vi "Periodic Tasks.vi"(8 "error in":errorcluster) -> ()   [LabVIEW 2020]
doc: "This VI runs in parallel to other tasks. It can contain as many user-defined periodic loops as you need. These can carry out PID or other sorts of timed response."
uses:
  <vilib>/Rock Robotics/WPI/ThirdParty/Sensors/navX/_TypeDefs/FRIC_navX_DeviceNumbersTypeDef.ctl
  <vilib>/Rock Robotics/WPI/ThirdParty/JAS_Junk/TrajLib/Rotation2d_CreateAngle.vi
  Robot Global Data.vi
  <vilib>/Rock Robotics/WPI/ThirdParty/Phoenix-LabVIEW/CANCoder/Get/CTRE_Phoenix_CANcoder_GetSensorData.vi
  <vilib>/Rock Robotics/WPI/ThirdParty/JAS_Junk/TrajLib/Trajectory_Library.lvlib
  <vilib>/Rock Robotics/Network Tables/NT Write Number.vi
  <vilib>/Rock Robotics/Network Tables/NT Write Boolean.vi
panel:
  out "POSE.TRANSLATION.Y":dbl
  out "POSE.TRANSLATION.X":dbl
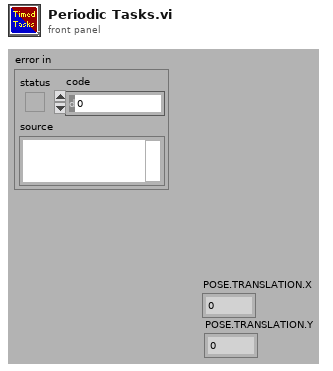
[diagram p1: front panel]
types:
  T1 = typedef "Trajectory_Library.lvlib/ROTATION2D.ctl" = cluster{"VALUE":dbl, "COS":dbl, "SIN":dbl}
  T2 = typedef "Trajectory_Library.lvlib/TRANSLATION2D.ctl" = cluster{"X":dbl, "Y":dbl}
  T3 = typedef "Trajectory_Library.lvlib/SWERVE_DRIVE_MODULE_POSITION.ctl" = cluster{"Distance":dbl, "Angle":T1, "P":bool}
  T4 = typedef "Trajectory_Library.lvlib/POSE2D.ctl" = cluster{"TRANSLATION":T2, "ROTATION":T1}
  T5 = typedef "Trajectory_Library.lvlib/SWERVE_DRIVE_KINEMATICS.ctl" = cluster{"NumModules":i32, "InverseKinematics":T6, "ForwardKinematics":T6, "Modules":T2[], "PrevCoR":T2, "SavedModuleStates":T7[]}
  T6 = typedef "NI_Matrix.lvlib/RealMatrix.ctl" = dbl[][]
  T7 = typedef "Trajectory_Library.lvlib/SWERVE_DRIVE_MODULE_STATE.ctl" = cluster{"Speed":dbl, "Angle":T1}
  T8 = typedef "Trajectory_Library.lvlib/SWERVE_DRIVE_ODOMETRY.ctl" = cluster{"POSE":T4, "GyroOffset":T1, "PreviousAngle":T1, "PrevModulePositions":T3[], "NumModules":i32}
  T9 = typedef "FRIC_navX_DeviceNumbersTypeDef.ctl" = enum16{"Dev0", "Dev1", "Dev2", "Dev3"}
  T10 = typedef "CTRE_Phoenix_CANcoder_DeviceRef.ctl" = cluster{"DeviceStatus":errorcluster, "Device Number":u8, "Handle":u64, "UsageFrame":u32, "Library Path":path}
  T11 = typedef "WPI_MotorControlDeviceRef.ctl" = cluster{"DeviceStatus":errorcluster, "Type":T12, "PWM":cluster{"PWM Channel":T13, "DeadBand":T14}, "CAN":cluster{"Device Number":u8, "SetOutput VI Ref":variant, "GetOutput VI Ref":variant, "Enable VI Ref":variant, "Disable VI Ref":variant, "Data":variant}, "Invert":bool, "DIO PWM":cluster{"PWM \"Enable\" Channel":T13, "DIOChannel":T15, "PWM Rate":dbl}}
  T12 = typedef "WPI_MotorControlType.ctl" = enum16{"PWM", "CAN", "DIO PWM"}
  T13 = typedef "FPGA_DIOPWMChannel.ctl" = enum8{"PWM 0", "PWM 1", "PWM 2", "PWM 3", "PWM 4", "PWM 5", "PWM 6", "PWM 7", "PWM 8", "PWM 9", "PWM MXP 0", "PWM MXP 1", "PWM MXP 2", "PWM MXP 3", "PWM MXP 4", "PWM MXP 5", "PWM MXP 6", "PWM MXP 7", "PWM MXP 8", "PWM MXP 9", "Invalid"}
  T14 = typedef "WPI_PWMDeadband.ctl" = cluster{"Name":string, "maxPositivePwm":i32, "minPositivePwm":i32, "centerPwm":i32, "maxNegativePwm":i32, "minNegativePwm":i32, "angularRange":u16}
  T15 = typedef "FPGA_DIOChannel.ctl" = enum8{"DIO 0", "DIO 1", "DIO 2", "DIO 3", "DIO 4", "DIO 5", "DIO 6", "DIO 7", "DIO 8", "DIO 9", "DIO MXP 0", "DIO MXP 1", "DIO MXP 2", "DIO MXP 3", "DIO MXP 4", "DIO MXP 5", "DIO MXP 6", "DIO MXP 7", "DIO MXP 8", "DIO MXP 9", "DIO MXP 10", "DIO MXP 11", "DIO MXP 12", "DIO MXP 13", "DIO MXP 14", "DIO MXP 15", "SPI Port CS1", "SPI Port CS2", "SPI Port CS3", "SPI Port MISO", "SPI Port MOSI", "Invalid"}
  T16 = cluster{"Yaw":dbl, "Roll":dbl, "Pitch":dbl, "Heading":dbl, "Fused Heading":dbl}
  T17 = cluster{"POSE.TRANSLATION.X":dbl, "POSE.TRANSLATION.Y":dbl}
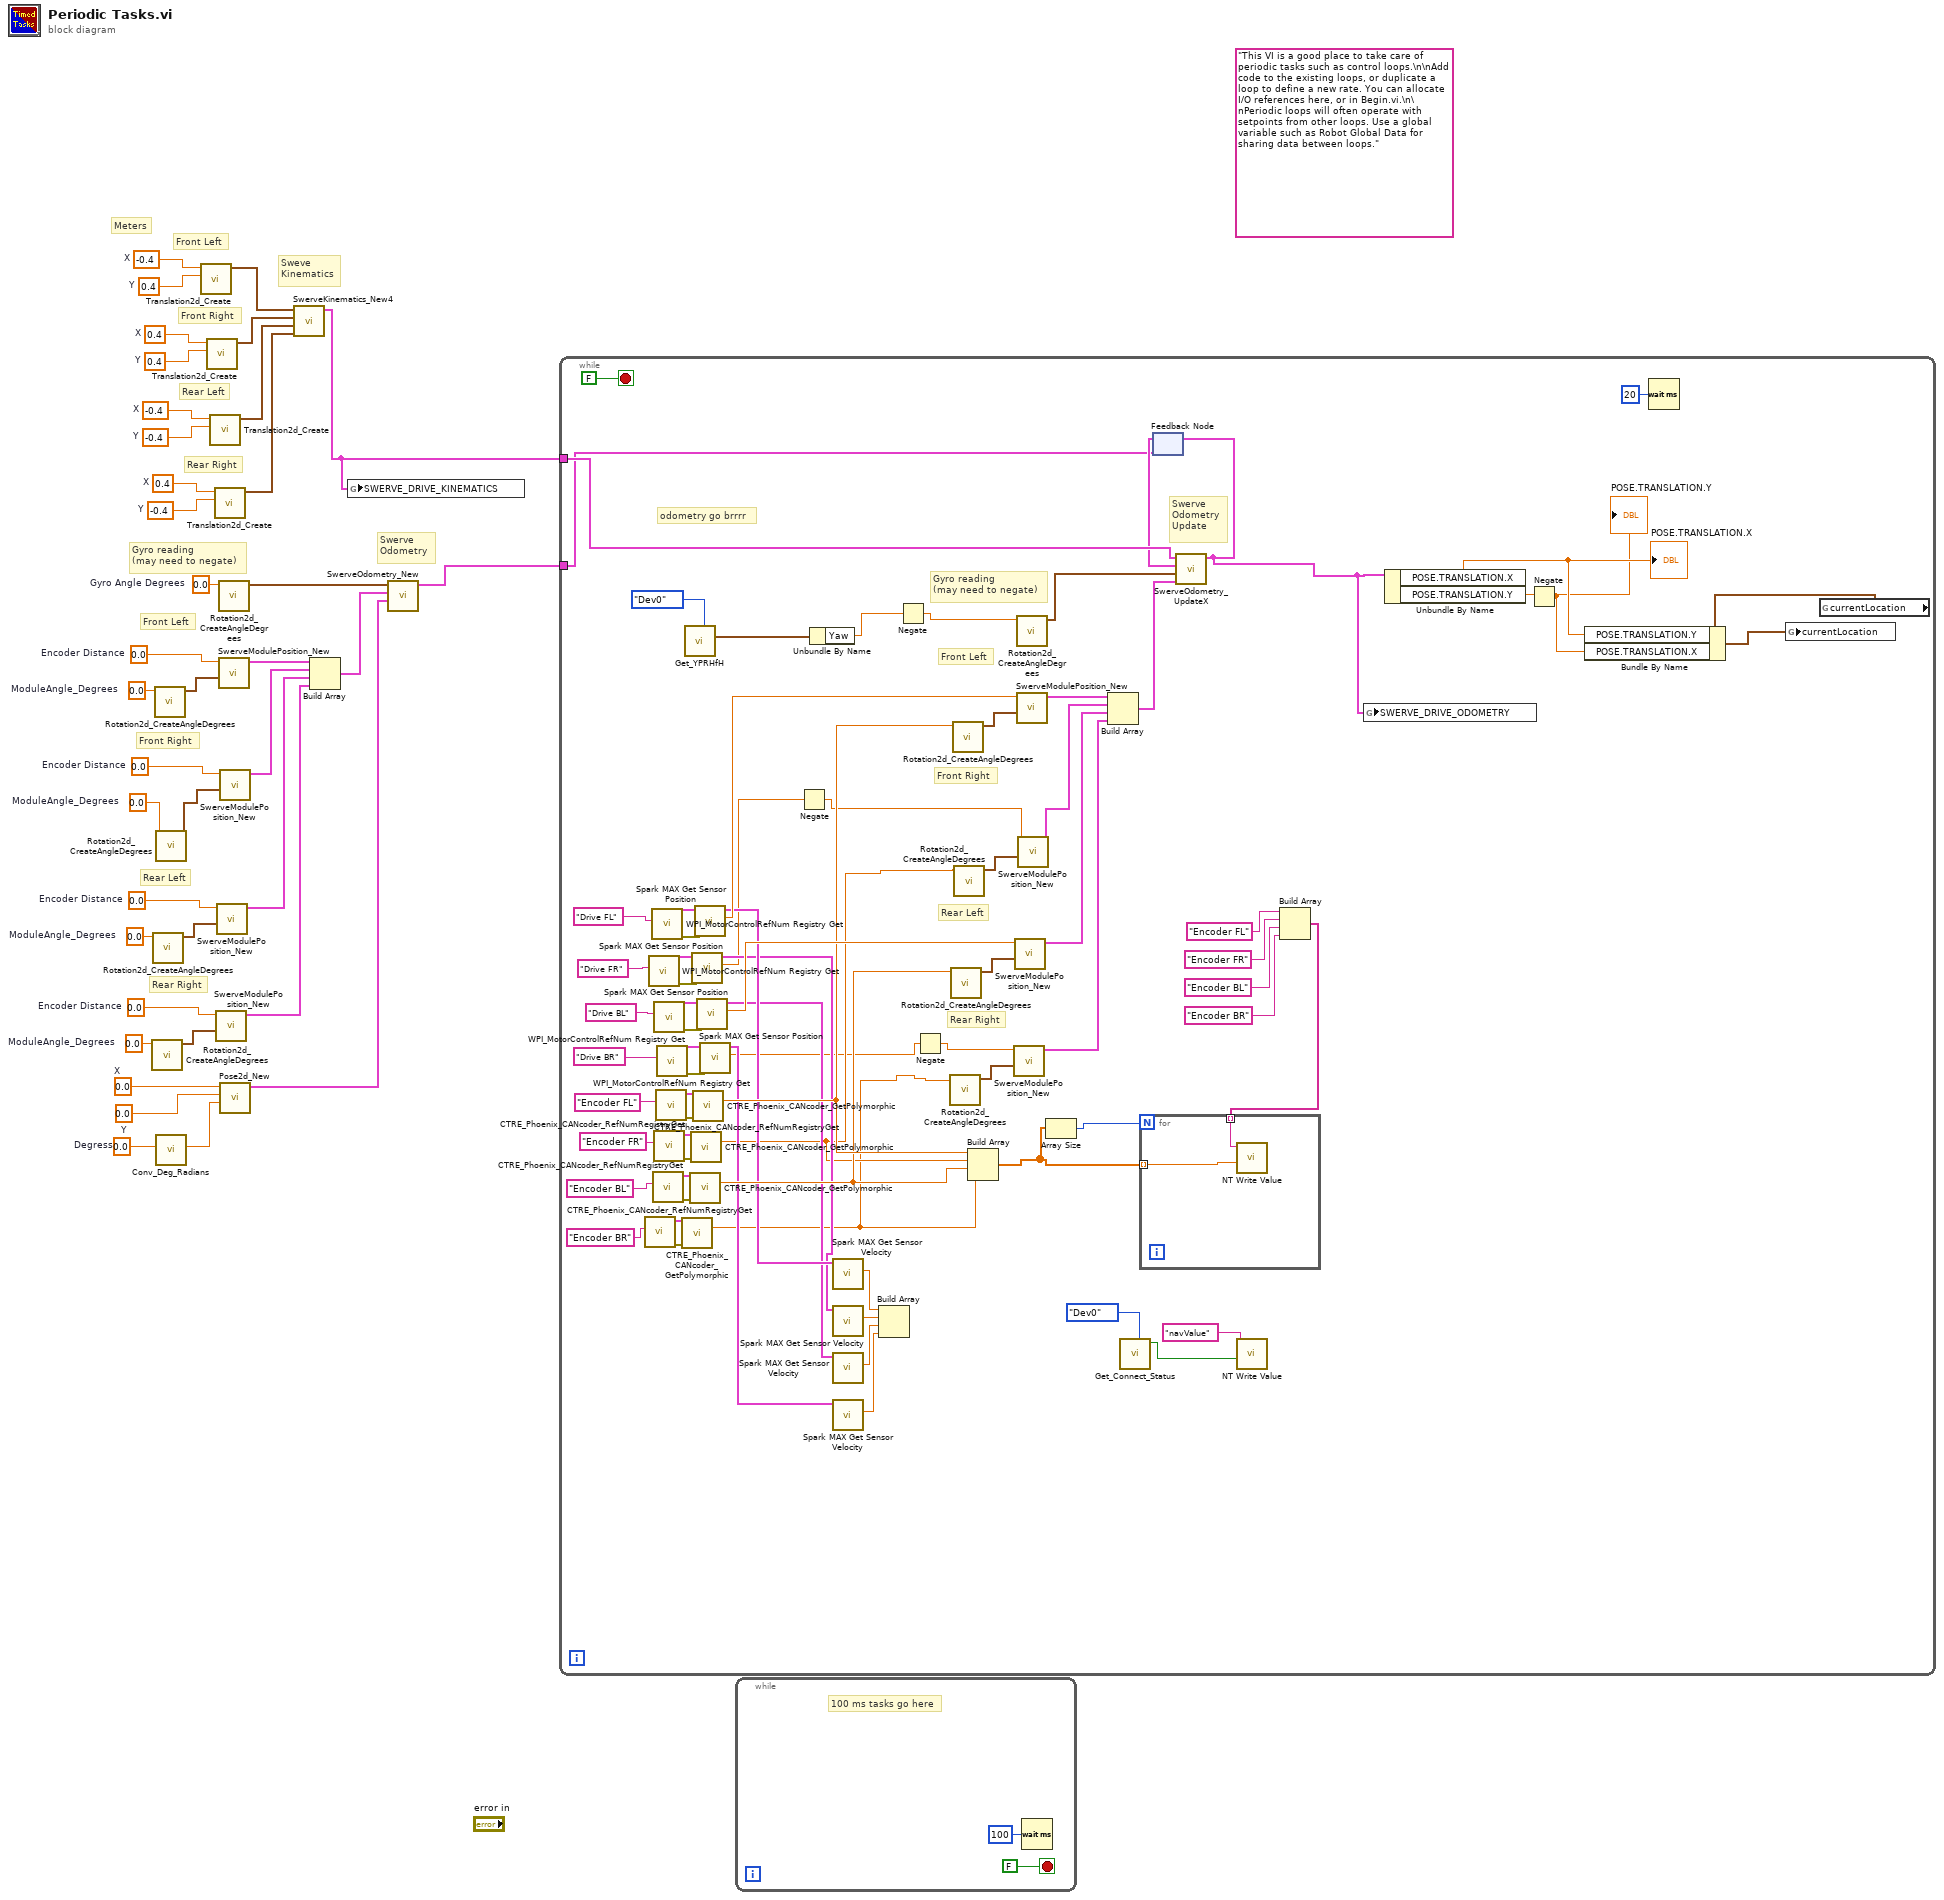
[diagram p0: block diagram]
diagram:
  w9 = 0.4  # X
  w8 = -0.4  # Y
  w7 = -0.4  # X
  w6 = -0.4  # Y
  w5 = 0.4  # X
  w4 = 0.4  # Y
  w3 = -0.4  # X
  w2 = 0.4  # Y
  w37 = 0.0  # Degress
  w36 = 0.0  # X
  w35 = 0.0  # Y
  w28 = 0.0  # ModuleAngle_Degrees
  w26 = 0.0  # Encoder Distance
  w25 = 0.0  # ModuleAngle_Degrees
  w23 = 0.0  # Encoder Distance
  w22 = 0.0  # ModuleAngle_Degrees
  w20 = 0.0  # Encoder Distance
  w18 = 0.0  # Gyro Angle Degrees
  w17 = 0.0  # ModuleAngle_Degrees
  w15 = 0.0  # Encoder Distance
  (unwired) "This VI is a good place to take care of periodic tasks such as control loops.\n\nAdd code to the existing loops, or duplicate a loop to define a new rate. You can allocate I/O references here, or in Begin.vi.\n\nPeriodic loops will often operate with setpoints from other loops. Use a global variable such as Robot Global Data for sharing data between loops."
  # "Meters"
  # "Sweve\nKinematics"
  # "Rear Right"
  # "Rear Left"
  # "Front Right"
  # "Front Left"
  # "Swerve\nOdometry"
  # "Rear Right"
  # "Rear Left"
  # "Front Right"
  # "Front Left"
  # "Gyro reading\n(may need to negate)"
  n1 = call <vilib>:"Rotation2d_CreateAngleDegrees.vi"("Angle_Degrees"=w28) -> ("ROTATION"=w27:T1)  [unwired: 10 in]
  n2 = call <vilib>:"Rotation2d_CreateAngleDegrees.vi"("Angle_Degrees"=w25) -> ("ROTATION"=w24:T1)  [unwired: 10 in]
  n3 = call <vilib>:"Rotation2d_CreateAngleDegrees.vi"("Angle_Degrees"=w17) -> ("ROTATION"=w16:T1)  [unwired: 10 in]
  n4 = call <vilib>:"Rotation2d_CreateAngleDegrees.vi"("Angle_Degrees"=w22) -> ("ROTATION"=w21:T1)  [unwired: 10 in]
  n5 = call <vilib>:"Conv_Deg_Radians.vi"("Degress"=w37) -> ("Radians"=w34:dbl)  [unwired: 10 in]
  n6 = call <vilib>:"Translation2d_Create.vi"("Y"=w2, "X"=w3) -> ("TRANSLATION"=w10:T2)  [unwired: 9 in]
  n7 = call <vilib>:"Translation2d_Create.vi"("Y"=w4, "X"=w5) -> ("TRANSLATION"=w11:T2)  [unwired: 9 in]
  n8 = call <vilib>:"Translation2d_Create.vi"("Y"=w6, "X"=w7) -> ("TRANSLATION"=w12:T2)  [unwired: 9 in]
  n9 = call <vilib>:"Translation2d_Create.vi"("Y"=w8, "X"=w9) -> ("TRANSLATION"=w13:T2)  [unwired: 9 in]
  n10 = call <vilib>:"SwerveModulePosition_New.vi"("ROTATION"=w27, "Distance"=w26) -> ("SWERVE_DRIVE_MODULE_POSITION"=w31:T3)  [unwired: 9 in]
  n11 = call <vilib>:"SwerveModulePosition_New.vi"("ROTATION"=w24, "Distance"=w23) -> ("SWERVE_DRIVE_MODULE_POSITION"=w30:T3)  [unwired: 9 in]
  n12 = call <vilib>:"Rotation2d_CreateAngleDegrees.vi"("Angle_Degrees"=w18) -> ("ROTATION"=w32:T1)  [unwired: 10 in]
  n13 = call <vilib>:"SwerveModulePosition_New.vi"("ROTATION"=w16, "Distance"=w15) -> ("SWERVE_DRIVE_MODULE_POSITION"=w19:T3)  [unwired: 9 in]
  n14 = call <vilib>:"SwerveModulePosition_New.vi"("ROTATION"=w21, "Distance"=w20) -> ("SWERVE_DRIVE_MODULE_POSITION"=w29:T3)  [unwired: 9 in]
  n15 = call <vilib>:"Pose2d_New.vi"("Heading"=w34, "Y"=w35, "X"=w36) -> ("out POSe"=w38:T4)  [unwired: 8 in]
  n16 = call <vilib>:"SwerveKinematics_New4.vi"("wheel 3"=w13, "wheel 2"=w12, "wheel 1"=w11, "wheel 0"=w10) -> ("SWERVE_DRIVE_KINEMATICS"=w1:T5)  [unwired: 7 in]
  n17 = Build Array(w19, w29, w30, w31) -> (w33:T3[])
  n18 = global write "Robot Global Data.vi" "SWERVE_DRIVE_KINEMATICS"(w1) -> ()
  n19 = call <vilib>:"SwerveOdometry_New.vi"("InitialPose"=w38, "Module Positions"=w33, "gyroAngle"=w32) -> ("SWERVE_DRIVE_ODOMETRY"=w14:T8)  [unwired: 8 in]
  n20 = while {
    tunnel: w14 -> [w61]
    tunnel: w1 -> [w73]
    stop <- FALSE stop-if-true
    # "Swerve\nOdometry\nUpdate"
    # "Rear Right"
    # "Rear Left"
    # "Front Right"
    # "Front Left"
    # "Gyro reading\n(may need to negate)"
    # "odometry go brrrr"
    n21 = call <vilib>:"CTRE_Phoenix_CANcoder_RefNumRegistryGet.vi"("refnum name"="Encoder BR") -> ("error out"=w96:errorcluster, "CTRE_CANcoder_DeviceRef"=w97:T10)  [unwired: 9 in]
    n22 = call <vilib>:"WPI_MotorControlRefNum Registry Get.vi"("refnum name"="Drive FR") -> ("error out"=w89:errorcluster, "MotorControlDevRef"=w88:T11)  [unwired: 9 in]
    n23 = call <vilib>:"WPI_MotorControlRefNum Registry Get.vi"("refnum name"="Drive FL") -> ("error out"=w91:errorcluster, "MotorControlDevRef"=w90:T11)  [unwired: 9 in]
    n24 = call <vilib>:"CTRE_Phoenix_CANcoder_RefNumRegistryGet.vi"("refnum name"="Encoder BL") -> ("error out"=w98:errorcluster, "CTRE_CANcoder_DeviceRef"=w99:T10)  [unwired: 9 in]
    n25 = call <vilib>:"WPI_MotorControlRefNum Registry Get.vi"("refnum name"="Drive BL") -> ("error out"=w87:errorcluster, "MotorControlDevRef"=w86:T11)  [unwired: 9 in]
    n26 = call <vilib>:"CTRE_Phoenix_CANcoder_RefNumRegistryGet.vi"("refnum name"="Encoder FR") -> ("error out"=w100:errorcluster, "CTRE_CANcoder_DeviceRef"=w101:T10)  [unwired: 9 in]
    n27 = call <vilib>:"CTRE_Phoenix_CANcoder_RefNumRegistryGet.vi"("refnum name"="Encoder FL") -> ("error out"=w102:errorcluster, "CTRE_CANcoder_DeviceRef"=w103:T10)  [unwired: 9 in]
    n28 = call <vilib>:"WPI_MotorControlRefNum Registry Get.vi"("refnum name"="Drive BR") -> ("error out"=w85:errorcluster, "MotorControlDevRef"=w84:T11)  [unwired: 9 in]
    n29 = call-poly <vilib>:"CTRE_Phoenix_CANcoder_GetPolymorphic.vi"("CTRE_CANcoder_DeviceRef"=w97, "error in"=w96) -> ("Position"=w58:dbl)  [unwired: 9 in, 4 out]
    n30 = call <vilib>:"Get_YPRHfH.vi"("Device Number"=FRIC_navX_DeviceNumbersTypeDef."Dev0") -> ("YRPHfH"=w104:T16)  [unwired: 10 in]
    n31 = call-poly <vilib>:"CTRE_Phoenix_CANcoder_GetPolymorphic.vi"("CTRE_CANcoder_DeviceRef"=w99, "error in"=w98) -> ("Position"=w71:dbl)  [unwired: 9 in, 4 out]
    n32 = call-poly <vilib>:"CTRE_Phoenix_CANcoder_GetPolymorphic.vi"("CTRE_CANcoder_DeviceRef"=w101, "error in"=w100) -> ("Position"=w59:dbl)  [unwired: 9 in, 4 out]
    n33 = call <vilib>:"Spark MAX Get Sensor Position.vi"("error in (no error)"=w89, "MotorControlDevRef in"=w88) -> ("Sensor Position"=w54:dbl, "MotorControlDevRef out"=w69:T11)  [unwired: 6 in, 2 out]
    n34 = call-poly <vilib>:"CTRE_Phoenix_CANcoder_GetPolymorphic.vi"("CTRE_CANcoder_DeviceRef"=w103, "error in"=w102) -> ("Position"=w72:dbl)  [unwired: 9 in, 4 out]
    n35 = call <vilib>:"Spark MAX Get Sensor Position.vi"("error in (no error)"=w91, "MotorControlDevRef in"=w90) -> ("Sensor Position"=w76:dbl, "MotorControlDevRef out"=w70:T11)  [unwired: 6 in, 2 out]
    n36 = call <vilib>:"Spark MAX Get Sensor Position.vi"("error in (no error)"=w87, "MotorControlDevRef in"=w86) -> ("Sensor Position"=w75:dbl, "MotorControlDevRef out"=w68:T11)  [unwired: 6 in, 2 out]
    n37 = call <vilib>:"Spark MAX Get Sensor Position.vi"("error in (no error)"=w85, "MotorControlDevRef in"=w84) -> ("Sensor Position"=w52:dbl, "MotorControlDevRef out"=w67:T11)  [unwired: 6 in, 2 out]
    n38 = Negate(x=w54) -> (-x=w53:dbl)
    n39 = Unbundle By Name(w104) -> ("Yaw"=w56:dbl)
    n40 = call <vilib>:"Spark MAX Get Sensor Velocity.vi"("MotorControlDevRef in"=w70) -> ("Sensor Velocity"=w66:dbl)  [unwired: 7 in, 3 out]
    n41 = call <vilib>:"Spark MAX Get Sensor Velocity.vi"("MotorControlDevRef in"=w69) -> ("Sensor Velocity"=w65:dbl)  [unwired: 7 in, 3 out]
    n42 = call <vilib>:"Spark MAX Get Sensor Velocity.vi"("MotorControlDevRef in"=w68) -> ("Sensor Velocity"=w64:dbl)  [unwired: 7 in, 3 out]
    n43 = call <vilib>:"Spark MAX Get Sensor Velocity.vi"("MotorControlDevRef in"=w67) -> ("Sensor Velocity"=w63:dbl)  [unwired: 7 in, 3 out]
    n44 = Build Array(w66, w65, w64, w63) -> ()  [unwired: 1 out]
    n45 = Negate(x=w56) -> (-x=w55:dbl)
    n46 = Negate(x=w52) -> (-x=w51:dbl)
    n47 = call <vilib>:"Rotation2d_CreateAngleDegrees.vi"("Angle_Degrees"=w58) -> ("ROTATION"=w110:T1)  [unwired: 10 in]
    n48 = call <vilib>:"Rotation2d_CreateAngleDegrees.vi"("Angle_Degrees"=w71) -> ("ROTATION"=w109:T1)  [unwired: 10 in]
    n49 = call <vilib>:"Rotation2d_CreateAngleDegrees.vi"("Angle_Degrees"=w72) -> ("ROTATION"=w106:T1)  [unwired: 10 in]
    n50 = call <vilib>:"Rotation2d_CreateAngleDegrees.vi"("Angle_Degrees"=w59) -> ("ROTATION"=w108:T1)  [unwired: 10 in]
    n51 = Build Array(w72, w59, w71, w58) -> (w47:dbl[])
    n52 = call <vilib>:"SwerveModulePosition_New.vi"("ROTATION"=w110, "Distance"=w51) -> ("SWERVE_DRIVE_MODULE_POSITION"=w113:T3)  [unwired: 9 in]
    n53 = call <vilib>:"SwerveModulePosition_New.vi"("ROTATION"=w109, "Distance"=w75) -> ("SWERVE_DRIVE_MODULE_POSITION"=w112:T3)  [unwired: 9 in]
    n54 = call <vilib>:"Rotation2d_CreateAngleDegrees.vi"("Angle_Degrees"=w55) -> ("ROTATION"=w57:T1)  [unwired: 10 in]
    n55 = call <vilib>:"SwerveModulePosition_New.vi"("ROTATION"=w106, "Distance"=w76) -> ("SWERVE_DRIVE_MODULE_POSITION"=w107:T3)  [unwired: 9 in]
    n56 = call <vilib>:"SwerveModulePosition_New.vi"("ROTATION"=w108, "Distance"=w53) -> ("SWERVE_DRIVE_MODULE_POSITION"=w111:T3)  [unwired: 9 in]
    n57 = Array Size(array=w47) -> (size(s)=w48:i32)
    n58 = Build Array(w107, w111, w112, w113) -> (w79:T3[])
    n59 = call <vilib>:"Get_Connect_Status.vi"("Device Number"=FRIC_navX_DeviceNumbersTypeDef."Dev0") -> ("Connected"=w41:bool)  [unwired: 10 in]
    n60 = feedback #1(w61) -> (w62:T8)
    n61 = call <vilib>:"SwerveOdometry_UpdateX.vi"("module Positions"=w79, "gyroAngle"=w57, "in SWERVE_DRIVE_ODOMETRY"=w62, "SWERVE_DRIVE_KINEMATICS"=w73) -> ("out SWERVE_DRIVE_ODOMETRY"=w60:T8)  [unwired: 5 in, 2 out]
    n62 = feedback-in #1(w60) -> ()
    n63 = call-poly <vilib>:"NT Write Value.vi"("value"=w41, "name"="navValue") -> ()  [unwired: 9 in, 1 out]
    n64 = Build Array("Encoder FL", "Encoder FR", "Encoder BL", "Encoder BR") -> (w42:string[])
    n65 = for {
      N: w48 -> [_]
      tunnel: w47 -> [w117] mode=indexing
      tunnel: w42 -> [w116] mode=indexing
      n66 = call-poly <vilib>:"NT Write Value.vi"("value"=w117, "name"=w116) -> ()  [unwired: 9 in, 1 out]
    }
    n67 = global write "Robot Global Data.vi" "SWERVE_DRIVE_ODOMETRY"(w60) -> ()
    n68 = Unbundle By Name(w60) -> ("POSE.TRANSLATION.X"=w74:dbl, "POSE.TRANSLATION.Y"=w50:dbl)
    "POSE.TRANSLATION.X" <- w74
    n69 = Negate(x=w50) -> (-x=w49:dbl)
    "POSE.TRANSLATION.Y" <- w49
    n70 = Wait (ms)(milliseconds to wait=u32 20) -> ()  [unwired: 1 out]
    n71 = global read "Robot Global Data.vi" "currentLocation"() -> (w77:T17)
    n72 = Bundle By Name(cluster=w77, "POSE.TRANSLATION.Y"=w74, "POSE.TRANSLATION.X"=w49) -> (w78:T17)
    n73 = global write "Robot Global Data.vi" "currentLocation"(w78) -> ()
  }
  n74 = while {
    stop <- FALSE stop-if-true
    # "100 ms tasks go here"
    n75 = Wait (ms)(milliseconds to wait=u32 100) -> ()  [unwired: 1 out]
  }
